vi "更新全局变量.vi"() -> ()   [LabVIEW 2016, in "update.lvlib"]
uses:
  update.lvlib
panel:
  out "MD5":string
  out "文件大小":i64
  out "已下载大小":i64
  out "滑动杆":dbl(slide) scale=0.0..100.0
  out "command":string caption="命令"
  out "last status string":string caption="最近状态字符串"
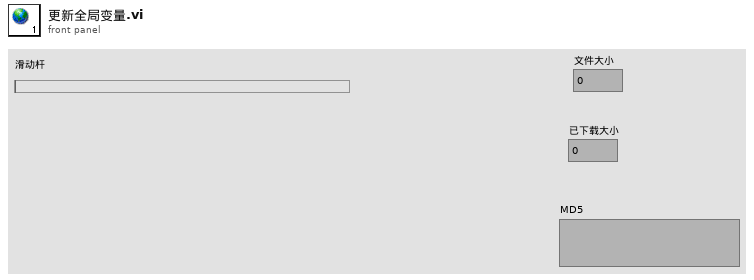
[diagram p1: front panel]
diagram:
